vi "test_geneXY_vizuXY.vi"() -> ()   [LabVIEW 2013]
uses:
  <vilib>/Analysis/Matrix/Datatypes/RealMatrix.ctl
  <vilib>/Analysis/Matrix/NI_Matrix.lvlib
panel:
  out "Graphe XY":T1(graph)
  out "final XY":T2
  in  "Number of Positions":u32=40
  in  "Spacing Y (µm)":dbl=0.1 step=0.001
  in  "Spacing X (µm)":dbl=0.1 step=0.001
  in  "Method":u8(ring) items=["Spiral Scan", "Column Scan", "Line Scan"]
  out "Field\nHeigth (µm)":dbl
  out "Field\nWidth (µm)":dbl
  in  "Microscope Objective\nMagnification":dbl=60.0 min=1.0 max=1000.0 step=1.0
  # "X"
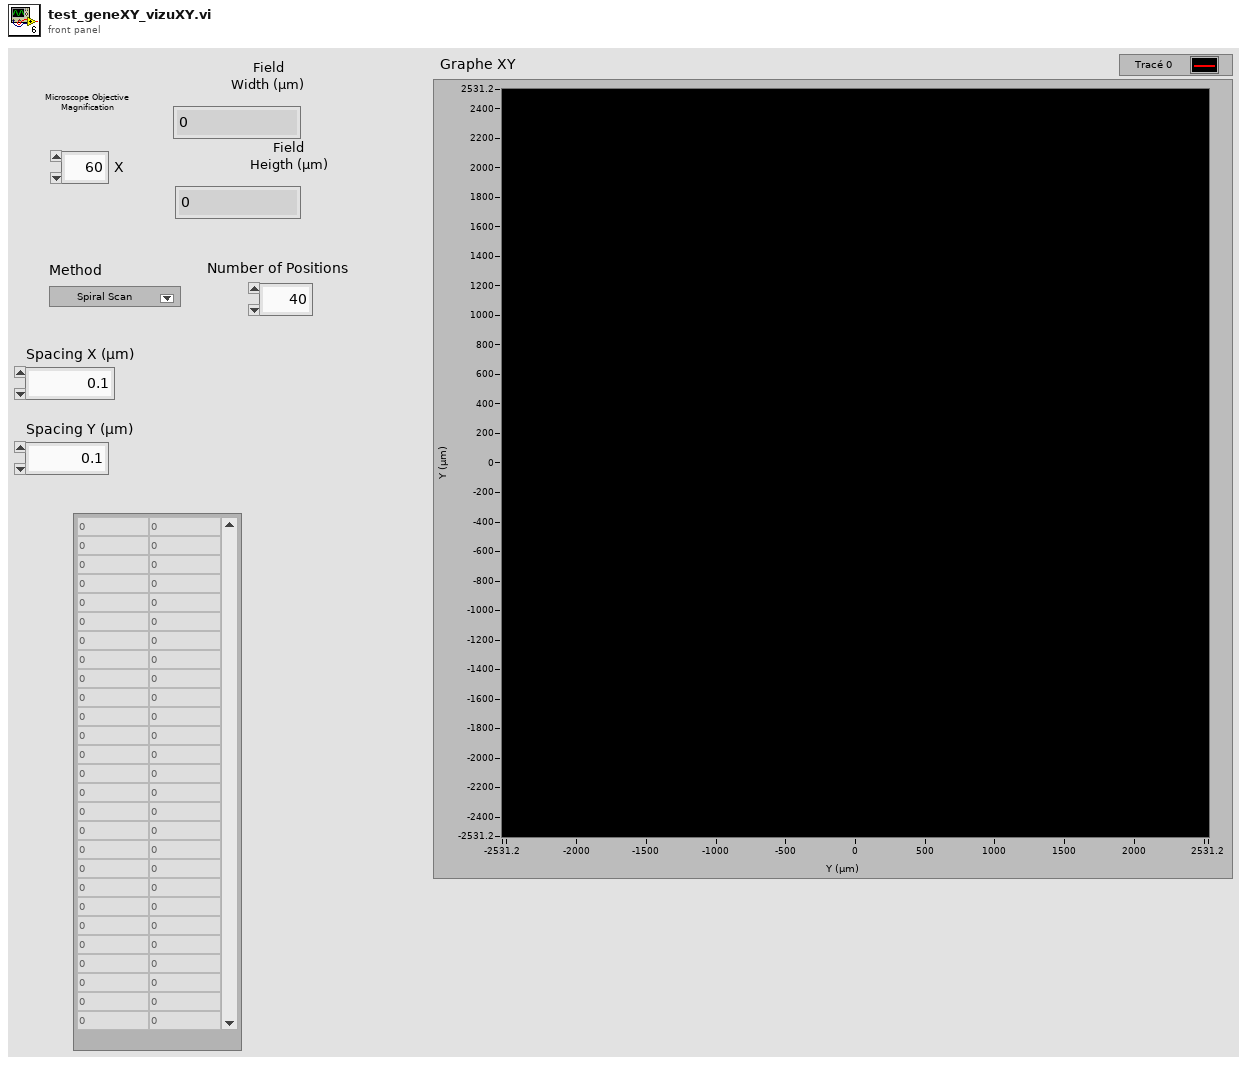
[diagram p1: front panel]
types:
  T1 = cluster{cluster{"Real Matrix Element":dbl, "Real Matrix Element":dbl}[]}[]
  T2 = typedef "NI_Matrix.lvlib/RealMatrix.ctl" = dbl[][]
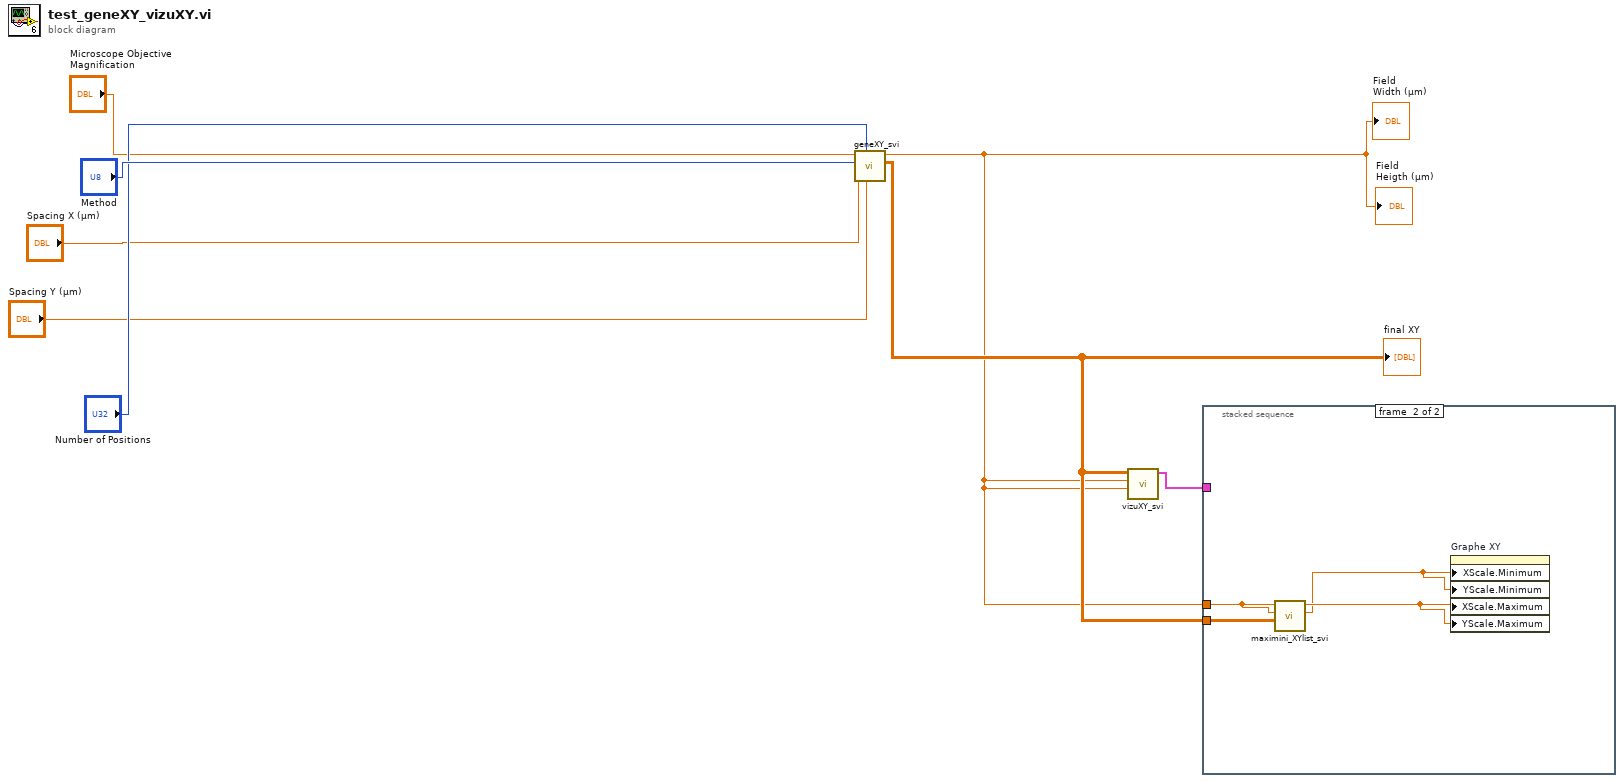
[diagram p0: block diagram]
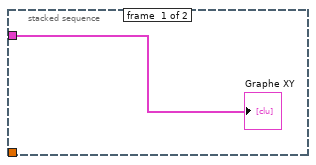
[diagram p2: hidden frame]
diagram:
  n1 = call "geneXY_svi.vi"("Spacing Y (µm)"="Spacing Y (µm)", "Number of Positions"="Number of Positions", "Spacing X (µm)"="Spacing X (µm)", "Method"="Method", "Microscope Objective\nMagnification"="Microscope Objective\nMagnification") -> ("Real Matrix"=w2:T2, "field_size(µm)"=w1:dbl)  [unwired: 5 in]
  "Field\nWidth (µm)" <- w1
  "Field\nHeigth (µm)" <- w1
  "final XY" <- w2
  n2 = call "vizuXY_svi.vi"("LY (mm)"=w1, "LX (mm)"=w1, "stored XY (µm)"=w2) -> ("Tableau"=w5:T1)  [unwired: 8 in]
  n3 = stacked-sequence {
    tunnel: w5 -> [w9 _]
    tunnel: w1 -> [_ w11]
    tunnel: w2 -> [_ w10]
    frame #0 {
      "Graphe XY" <- w9
    }
    frame #1 {
      n4 = call "maximini_XYlist_svi.vi"("stored XY"=w10, "LY"=w11, "LX"=w11) -> ("mini (µm)"=w12:dbl, "maxi (µm)"=w13:dbl)  [unwired: 7 in]
      n5 = property on="Graphe XY" class="GraphXY (strict)"("XScale.Minimum"=w12, "YScale.Minimum"=w12, "XScale.Maximum"=w13, "YScale.Maximum"=w13) -> ()  [unwired: 2 in, 2 out]
    }
  }
